vi "emballage nouvelle série_GPAO.vi"(1 "CodeBarFix":string, 2 "Nom du produit":string="12-216E-01-25 F120023 500mA 10Ohm", 3 "error in (no error)":errorcluster caption="entrée d'erreur (pas d'erreur)", 6 "Verif.Indice Client":bool) -> (5 "error out":errorcluster caption="sortie d'erreur", 11 "Indice Client":string, 14 "No commande FAS":string, 16 "DATA cmde":T1={"n°article FAS"="12-216E-01-25 F120023 500mA 10ohm", "n° cmde FAS"="R03844/08-01.01.01", "quantité cmde"="4", "ID LIG cmde"="225540", "n° cmde client"="120565              ", "nom client"="Fluid Automat. Systems GmbH", "n° article client"="21088", "indice revision client"="      ", "société de facturation"="FAS Medic SA                            ", "langue a utiliser"="ALL"}, 17 "Quantité de la commande":string="4", 18 "Commande interne":bool, 19 "Annuler(T=OK)":bool)   [LabVIEW 2020]
uses:
  Modules/FS/60_FS_Controles/60_FS_SetGet.ctl
  VG_VerifTests_ModeRetour.vi
panel:
  out "Cde_GPAO":bool
  in  "Cmde_Interne?":bool
  out "Indice Piece":string
  out "Tableau historique":string[][](array[string])=[["112105740008090004", "01.01.2001 01:01:00", "55", "01234/08-01.01.01", "1", "0"], ["112105740008090006", "01.01.2001 01:01:00", "55", "56789/08-01.01.01", "3", "0"], ["112105740008090007", "01.01.2001 01:01:00", "55", "56789/08-01.01.01", "4", "0"], ["112105740008090007", "01.01.2001 01:01:00", "55", "00123/08-01.01.01", "2", "1"]]
  out "Glissière 2":u8(slide)=100 caption="Identification terminé." scale=0.0..100.0
  in  "Valider qtté":bool
  in  "modifier qtté":bool
  in  "Numéro de commande FAS":string(combo)
  in  "Valider cmde":bool
  in  "Annuler?":bool
  # "La recherche se fait uniquement avec le numéro d'article et du numéro de file.\nLa designation (24V,...) n'est pas tenue compte (sauf pour les Flatprop) !!"
  # "Numéro de commande FAS"
  # "Seul un responsable peut valider une commande R (Retour)"
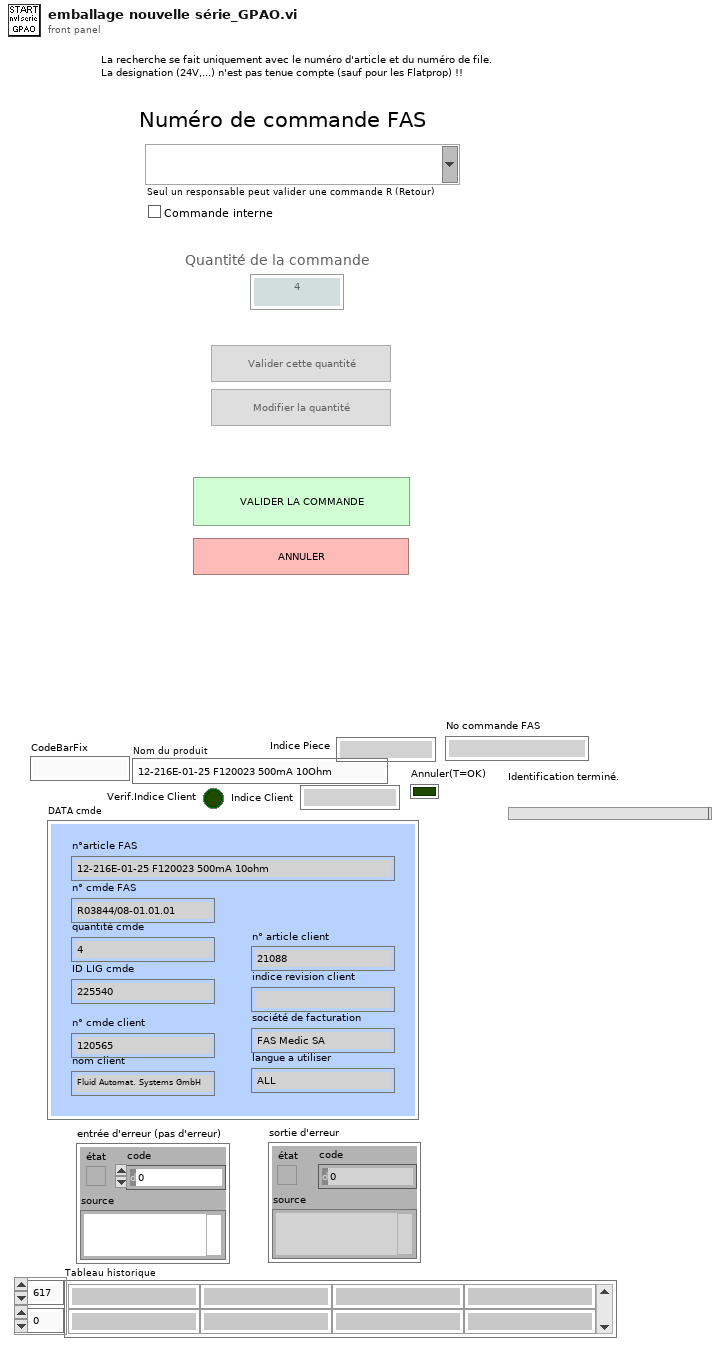
[diagram p1: front panel]
types:
  T1 = typedef "DATA commande.ctl" = cluster{"n°article FAS":string, "n° cmde FAS":string, "quantité cmde":string, "ID LIG cmde":string, "n° cmde client":string, "nom client":string, "n° article client":string, "indice revision client":string, "société de facturation":string, "langue a utiliser":string}
  T2 = typedef "60_FS_SetGet.ctl" = enum16{"set", "get"}
  T3 = enum16{"n° produit", "date", "opérateur", "n° cmde", "n° carton"}
  T4 = typedef "Emballage_BDD_param_Produit.ctl" = cluster{"No_Valve_FAS":string, "suffixe":string, "designation":string, "indice_produit":string, "code_barre_fixe":string, "affiche_code_barre_client":string, "affiche_no_client":string, "Nb_vlve_par_carton":u16, "melange_des_lots_possible":string, "id_article":string, "Indice_Rev":string, "Famille":string, "date":string, "code_barre_fixe_Fin":string, "Longeur_No_Serie":string}
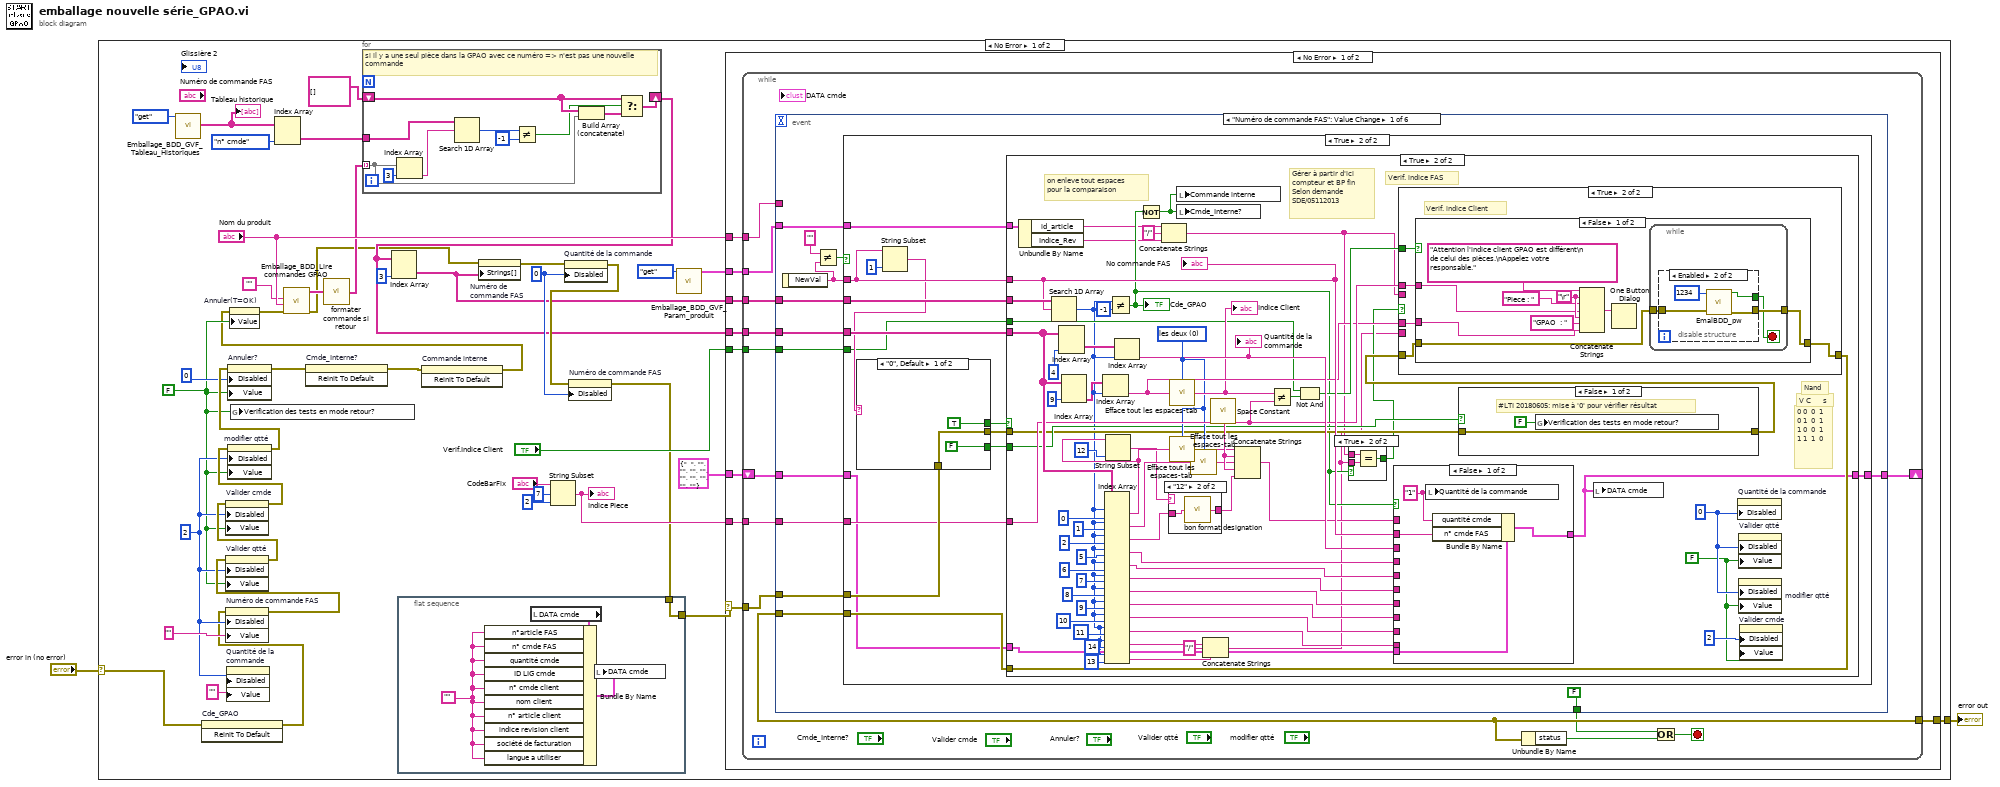
[diagram p0: block diagram]
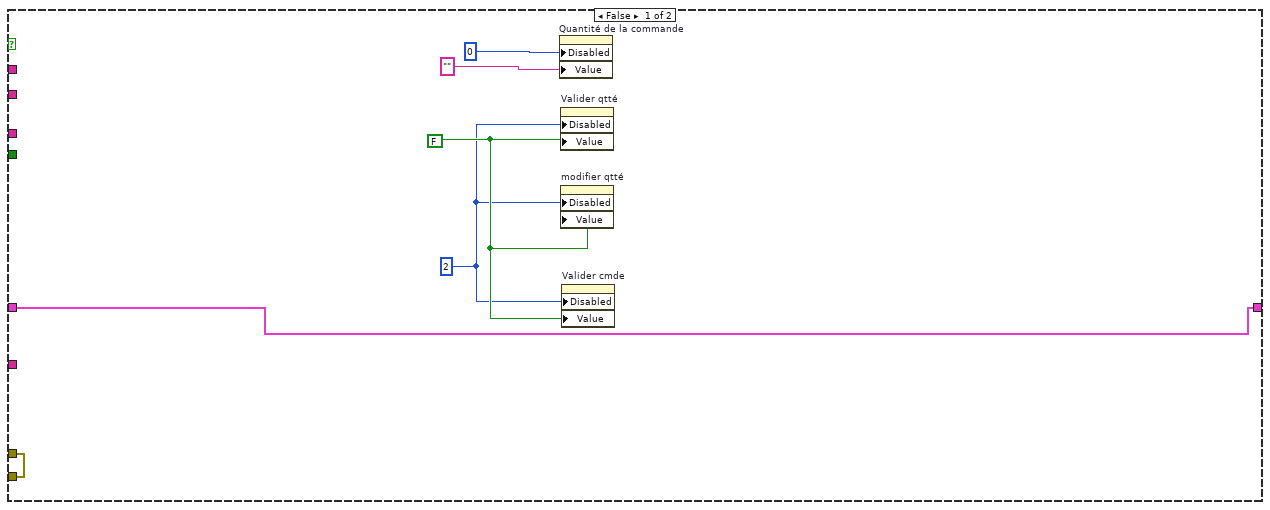
[diagram p2: hidden frame]
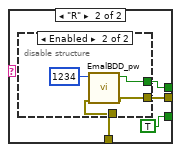
[diagram p3: hidden frame]
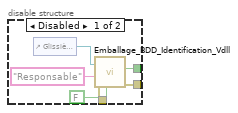
[diagram p4: hidden frame]
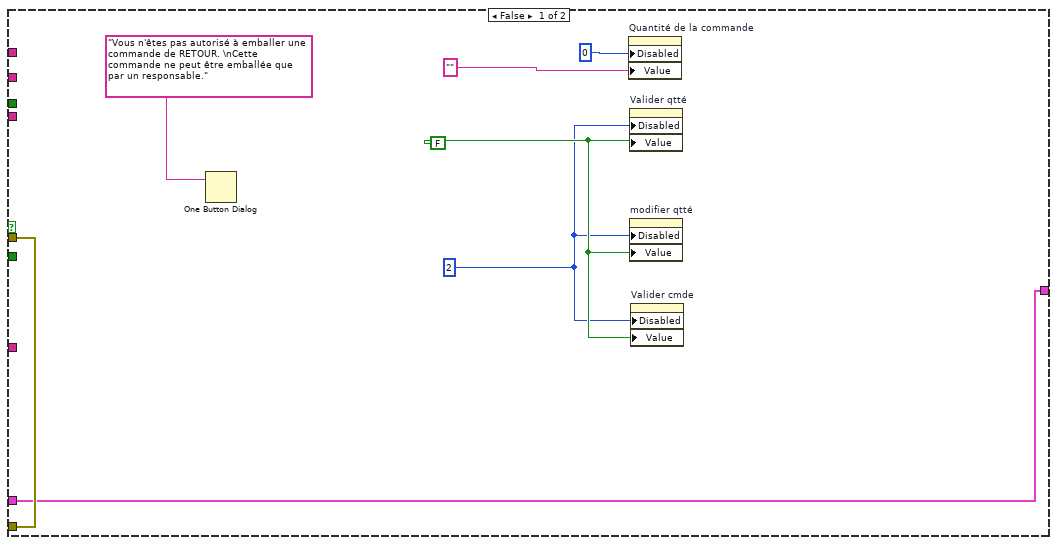
[diagram p5: hidden frame]
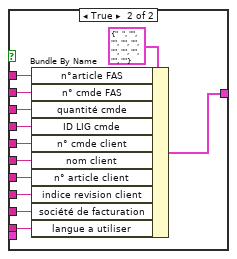
[diagram p6: hidden frame]
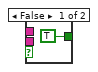
[diagram p7: hidden frame]
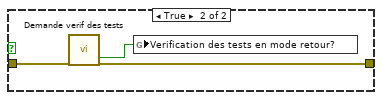
[diagram p8: hidden frame]
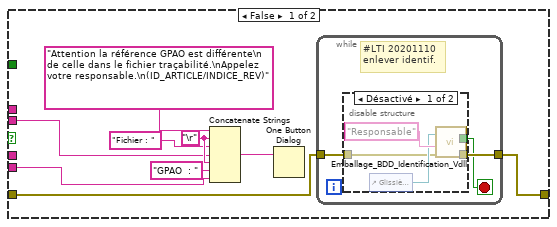
[diagram p9: hidden frame]
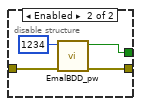
[diagram p10: hidden frame]
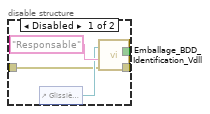
[diagram p11: hidden frame]
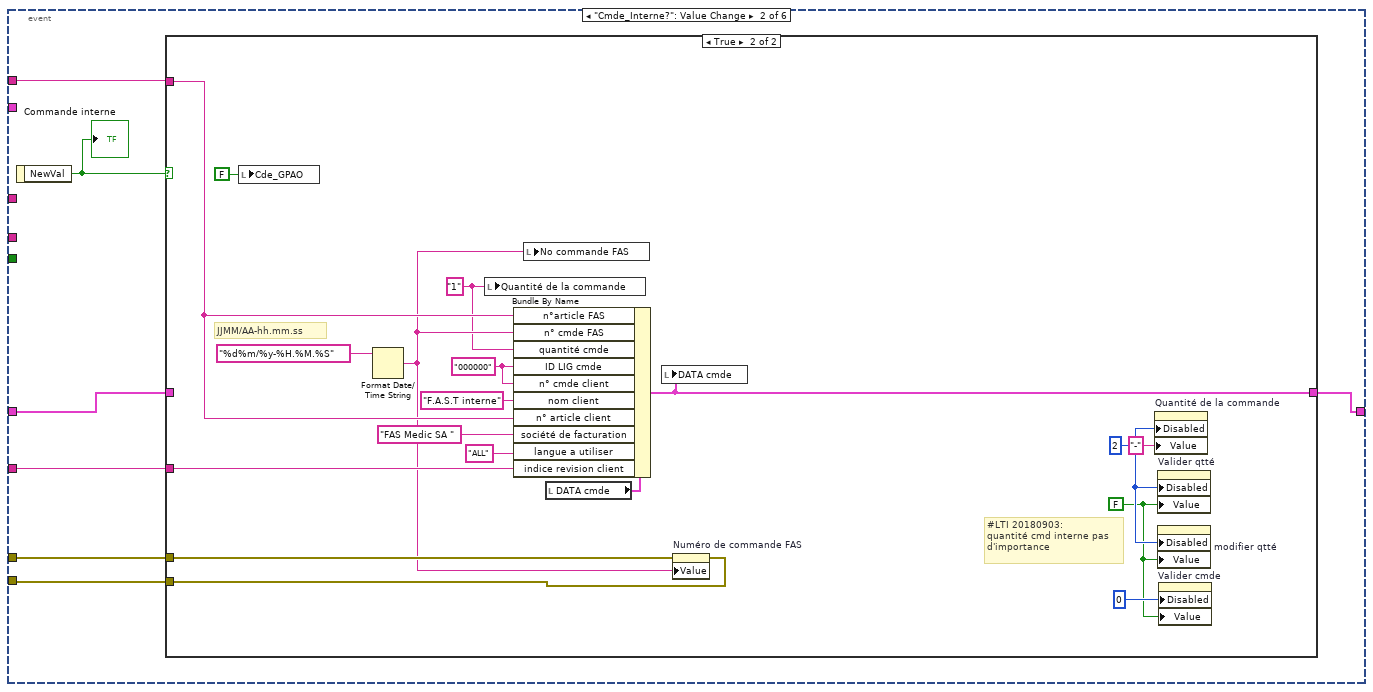
[diagram p14: hidden frame]
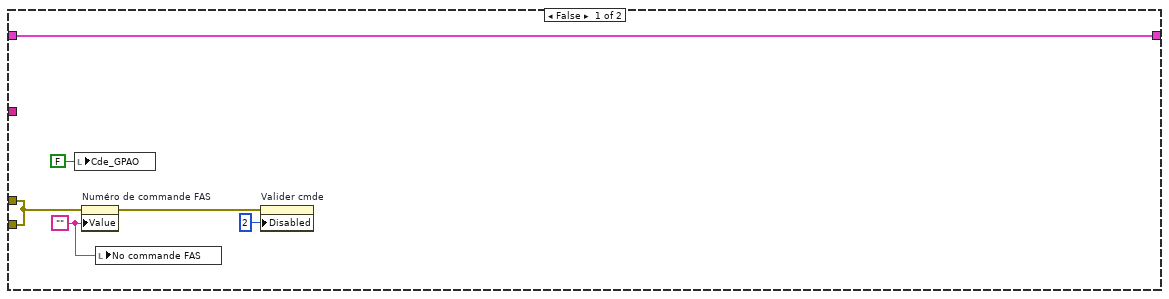
[diagram p15: hidden frame]
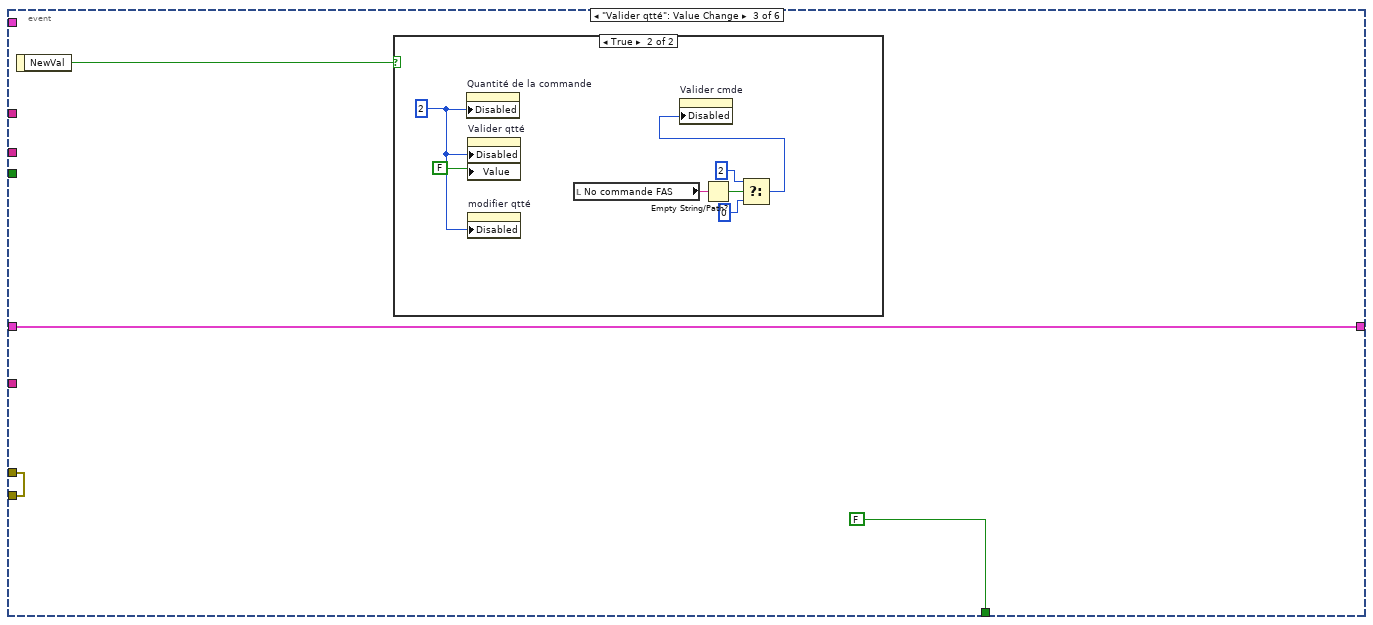
[diagram p16: hidden frame]
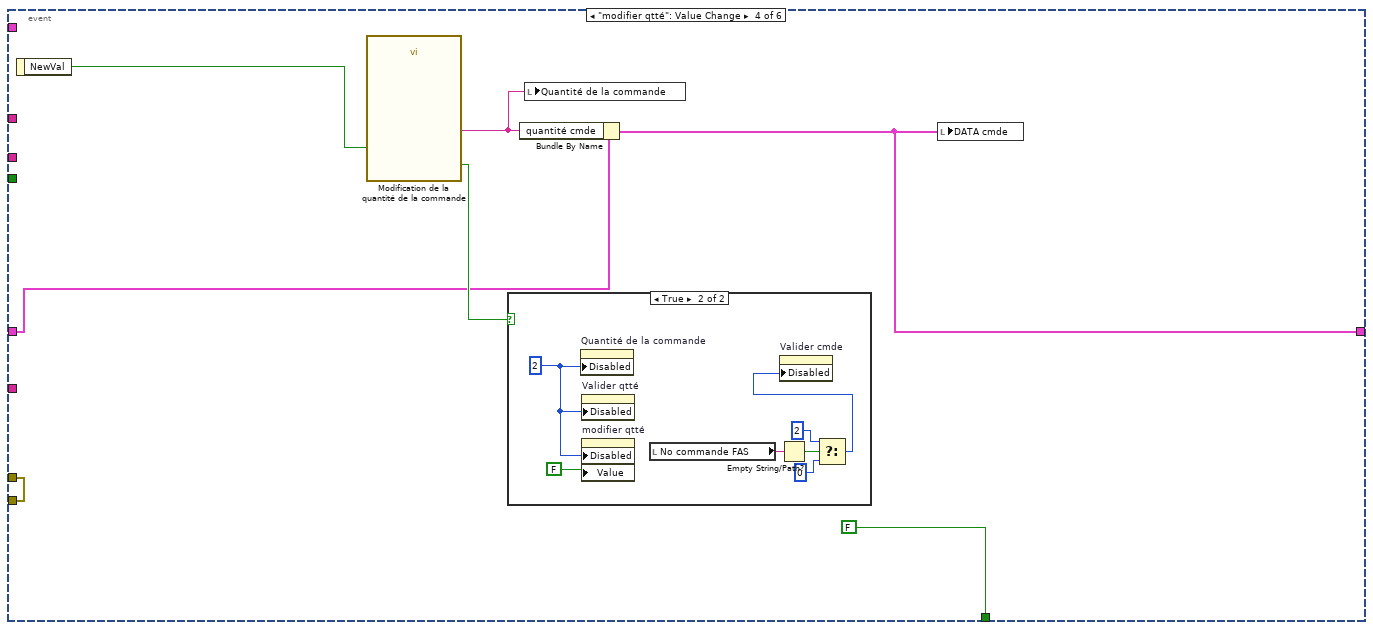
[diagram p18: hidden frame]
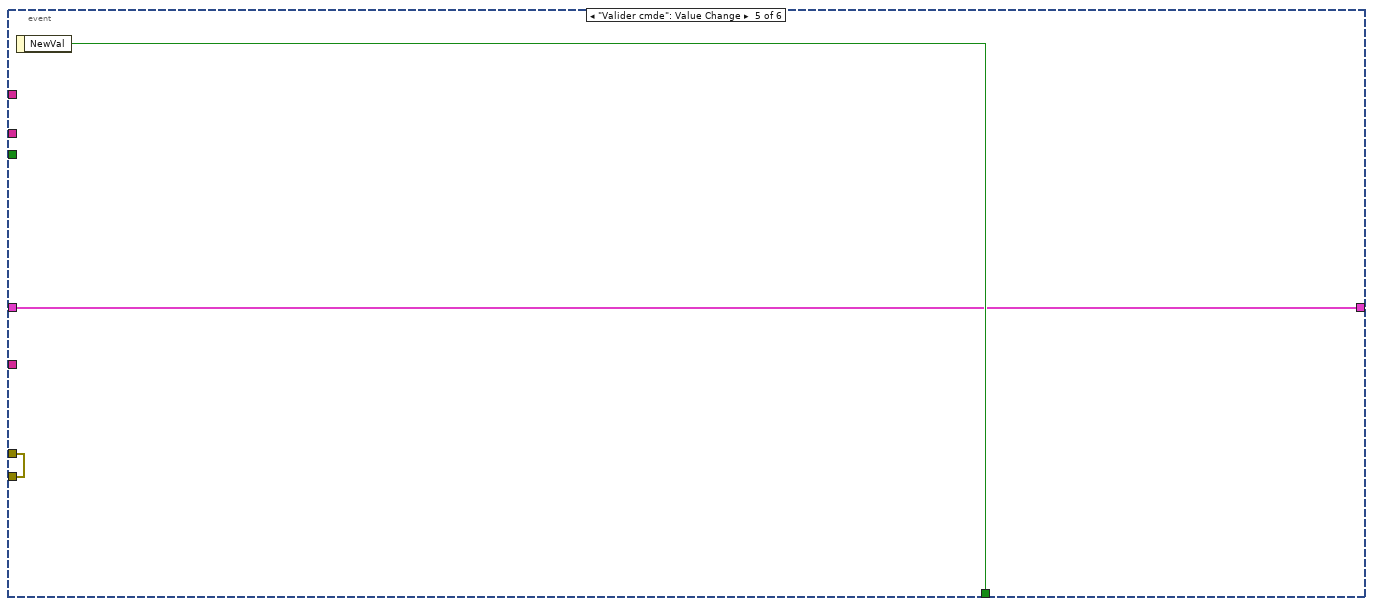
[diagram p20: hidden frame]
diagram:
  n1 = case shown="No Error" "error in (no error)" {
    selector: "error in (no error)" -> [w9 w350]
    tunnel: [w29 w350] -> w1
    frame No Error {
      w35 = u8 0 ("Désactivé")
      w39 = u8 2 ("Désactivé")
      w14 = FALSE
      n2 = call "Emballage_BDD_GVF_Tableau_Historiques.vi"("SetGet"=60_FS_SetGet."get") -> ("Tableau historique OUT"=w6:string[][])  [unwired: 9 in, 1 out]
      "Tableau historique" <- w6
      n3 = invoke on="Cde_GPAO" class="Bool (strict)" method="Reinit To Default"(error in=w9) -> (error out=w8:errorcluster)  [unwired: 2 in, 2 out]
      n4 = property on="Numéro de commande FAS" class="CmbBox"(error in=w8, "Disabled"=w39, "Value"="" ("Numéro de commande FAS")) -> (error out=w44:errorcluster)  [unwired: 1 in, 1 out]
      n5 = property on="Valider qtté" class="Bool (strict)"(error in=w44, "Disabled"=w39, "Value"=w14) -> (error out=w43:errorcluster)  [unwired: 1 in, 1 out]
      n6 = property on="Valider cmde" class="Bool (strict)"(error in=w43, "Disabled"=w39, "Value"=w14) -> (error out=w41:errorcluster)  [unwired: 1 in, 1 out]
      n7 = property on="Quantité de la commande" class="Str"("Disabled"=w39, "Value"="" ("Quantité de la commande")) -> ()  [unwired: 2 in, 2 out]
      n8 = property on="modifier qtté" class="Bool (strict)"(error in=w41, "Disabled"=w39, "Value"=w14) -> (error out=w40:errorcluster)  [unwired: 1 in, 1 out]
      n9 = property on="Annuler?" class="Bool (strict)"(error in=w40, "Disabled"=u8 0 ("Désactivé"), "Value"=w14) -> (error out=w13:errorcluster)  [unwired: 1 in, 1 out]
      n10 = global write "VG_VerifTests_ModeRetour.vi" "Verification des tests en mode retour?"(w14) -> ()
      n11 = Index Array(array=w6, index (col)=T3."n° cmde" ("Filtre")) -> (element=w26:string[])  [unwired: 1 in]
      n12 = invoke on="Cmde_Interne?" class="Bool (strict)" method="Reinit To Default"(error in=w13) -> (error out=w12:errorcluster)  [unwired: 2 in, 2 out]
      n13 = flat-sequence {
        tunnel: w10 -> [w345]
        tunnel: [w345] -> w30
        frame #0 {
          w344 = ""
          n14 = local read "DATA cmde"() -> (w347:T1)
          n15 = Bundle By Name(cluster=w347, "n°article FAS"=w344, "n° cmde FAS"=w344, "quantité cmde"=w344, "ID LIG cmde"=w344, "n° cmde client"=w344, "nom client"=w344, "n° article client"=w344, "indice revision client"=w344, "société de facturation"=w344, "langue a utiliser"=w344) -> (w346:T1)
          n16 = local write "DATA cmde"(w346) -> ()
        }
      }
      n17 = invoke on="Commande interne" class="Bool (strict)" method="Reinit To Default"(error in=w12) -> (error out=w11:errorcluster)  [unwired: 2 in, 2 out]
      n18 = property on="Annuler(T=OK)" class="Bool (strict)"(error in=w11, "Value"=w14) -> (error out=w33:errorcluster)  [unwired: 1 in, 1 out]
      n19 = call "Emballage_BDD_Lire  commandes GPAO.vi"("error in"=w33, "article"="Nom du produit", "Numéro commande"="") -> ("error out"=w21:errorcluster, "Tab cmde GPAO"=w31:string[][])  [unwired: 3 in, 4 out]
      n20 = call "formater commande si retour.vi"("Tab cmde GPAO IN"=w31) -> ("Tab cmde GPAO OUT"=w24:string[][])
      n21 = for {
        tunnel: w26 -> [w49]
        shift-right: [w54] -> w22
        shift-left: string[][] [] -> [w53]
        tunnel: w24 -> [w50] mode=indexing
        # "si il y a une seul pièce dans la GPAO avec ce numéro => n'est pas une nouvelle\ncommande"
        n22 = Index Array(array=w50, index=3 ("indice désactivé (col)")) -> (element=w48:string)
        n23 = Search 1D Array(1D array=w49, element=w48) -> (index of element=w47:i32)  [unwired: 1 in]
        n24 = Not Equal?(x=w47, y=-1) -> (x != y?=w45:bool)
        n25 = Build Array (concatenate)(w53, w50) -> (w52:string[][])
        n26 = Select(t=w53, s=w45, f=w52) -> (s? t:f=w54:string[][])
      }
      n27 = Index Array(array=w22, index (col)=3 ("indice désactivé (col)")) -> (element=w23:string[])  [unwired: 1 in]
      n28 = property on="Numéro de \ncommande FAS" class="CmbBox"(error in=w21, "Strings[]"=w23) -> (error out=w36:errorcluster)  [unwired: 1 in, 1 out]
      n29 = String Subset(string="CodeBarFix", offset (0)=7, length (rest)=2 ("longueur (reste)")) -> (substring=w16:string)
      "Indice Piece" <- w16
      n30 = property on="Quantité de la commande" class="Str"(error in=w36, "Disabled"=w35) -> (error out=w37:errorcluster)  [unwired: 1 in, 1 out]
      n31 = property on="Numéro de commande FAS" class="CmbBox"(error in=w37, "Disabled"=w35) -> (error out=w10:errorcluster)  [unwired: 1 in, 1 out]
      n32 = call "Emballage_BDD_GVF_Param_produit.vi"("Énum"=enum16{"set", "get"}."get") -> ("CLS_param_produit"=w3:T4)  [unwired: 7 in, 3 out]
      n33 = case shown="No Error" w30 {
        selector: w30 -> [w60 w343]
        tunnel: w23 -> [w63 _]
        tunnel: w22 -> [w62 _]
        tunnel: [w61 w343] -> w29
        tunnel: "Nom du produit" -> [w59 _]
        tunnel: w16 -> [w58 _]
        tunnel: "Verif.Indice Client" -> [w57 _]
        tunnel: T1 {"n°article FAS"="  ", "n° cmde FAS"="", "quantité cmde"="", "ID LIG cmde"="", "n° cmde client"="", "nom client"="", "n° article client"="", "indice revision client"="", "société de facturation"="", "langue a utiliser"=""} ("DATA cmde") -> [w56 _]
        tunnel: w3 -> [w55 _]
        frame No Error {
          n34 = while {
            tunnel: w63 -> [w76]
            tunnel: w62 -> [w75]
            tunnel: [w72] -> w61
            tunnel: w60 -> [w73]
            tunnel: w59 -> [w74]
            tunnel: w58 -> [w68]
            tunnel: w57 -> [w67]
            shift-right: [w66] -> _
            shift-left: w56 -> [w65]
            tunnel: w55 -> [w64]
            stop <- w71 stop-if-true
            n35 = event shown="[0] \"Numéro de commande FAS\": Value Change" {
              selector: _ -> [_ _ _ _ _ _]
              dyn-events: _ -> [_ _ _ _ _ _]
              timeout: _ -> [_ _ _ _ _ _]
              tunnel: w76 -> [w89 _ _ _ _ _]
              tunnel: w75 -> [w87 _ _ _ _ _]
              tunnel: [FALSE _ FALSE FALSE w336 w340] -> w70
              tunnel: w74 -> [_ w281 _ _ _ _]
              tunnel: w73 -> [w83 w283 w310 w322 w335 w338]
              tunnel: [w82 w282 w310 w322 w335 w338] -> w72
              tunnel: w68 -> [w81 w280 _ _ _ _]
              tunnel: w67 -> [w80 _ _ _ _ _]
              tunnel: [w79 w279 w309 w320 w334 w337] -> w66
              tunnel: w65 -> [w78 w278 w309 w321 w334 _]
              tunnel: w64 -> [w77 _ _ _ _ _]
              event "Numéro de commande FAS": Value Change {
                n36 = event-data() -> ("NewVal"=w84:string)  [unwired: 1 in]
                n37 = Not Equal?(x="" ("nouvel élément/sous-tableau"), y=w84) -> (x != y?=w86:bool)
                n38 = case shown="True" w86 {
                  tunnel: w89 -> [_ w110]
                  tunnel: w84 -> [_ w108]
                  tunnel: w87 -> [_ w109]
                  tunnel: w83 -> [w91 w104]
                  tunnel: [w91 w102] -> w82
                  tunnel: w81 -> [_ w101]
                  tunnel: w80 -> [_ w100]
                  tunnel: [w90 w98] -> w79
                  tunnel: w78 -> [w90 w97]
                  tunnel: w77 -> [_ w96]
                  frame False {
                    w95 = FALSE
                    w92 = u8 2 ("Désactivé")
                    n39 = property on="Quantité de la commande" class="Str"("Disabled"=u8 0 ("Désactivé"), "Value"="" ("nouvel élément/sous-tableau")) -> ()  [unwired: 2 in, 2 out]
                    n40 = property on="Valider qtté" class="Bool (strict)"("Disabled"=w92, "Value"=w95) -> ()  [unwired: 2 in, 2 out]
                    n41 = property on="modifier qtté" class="Bool (strict)"("Disabled"=w92, "Value"=w95) -> ()  [unwired: 2 in, 2 out]
                    n42 = property on="Valider cmde" class="Bool (strict)"("Disabled"=w92, "Value"=w95) -> ()  [unwired: 2 in, 2 out]
                  }
                  frame True {
                    n43 = String Subset(string=w108, length (rest)=1 ("longueur (reste)")) -> (substring=w106:string)  [unwired: 1 in]
                    n44 = case shown="\"0\", Default" w106 {
                      tunnel: [TRUE w116] -> w105
                      tunnel: w104 -> [w112 w117]
                      tunnel: [w112 w115] -> w103
                      tunnel: [FALSE ("lecture seul possible ?") TRUE ("lecture seul possible ?")] -> w99
                      frame "0", Default {
                      }
                      frame "R" {
                        n45 = disable-structure shown="Enabled" {
                          disable-tunnel: w117 -> [w121 w126]
                          disable-tunnel: [w120 w125] -> w116
                          disable-tunnel: [w118 w127] -> w115
                          frame Disabled {
                            n46 = control-ref of="Glissière 2"() -> (w119:refnum<vi>)
                            n47 = call "Emballage_BDD_Identification_Vdll.vi"("Glissière"=w119, "lecture seul possible ?"=FALSE, "error in"=w121, "Posage choisi"="Responsable") -> ("error Out"=w118:errorcluster, "OK"=w120:bool)  [unwired: 3 in, 3 out]
                          }
                          frame Enabled {
                            n48 = call "EmalBDD_pw.vi"("Error in"=w126, "PWattendu"=u32 1234) -> ("Error Out"=w127:errorcluster, "pwOK?"=w125:bool)  [unwired: 8 in]
                          }
                        }
                      }
                    }
                    n49 = case shown="True" w105 {
                      tunnel: w110 -> [_ w201]
                      tunnel: w108 -> [_ w193]
                      tunnel: w109 -> [_ w165]
                      tunnel: w103 -> [w129 w154]
                      tunnel: [w129 w166] -> w102
                      tunnel: w101 -> [_ w160]
                      tunnel: w100 -> [_ w147]
                      tunnel: w99 -> [_ w155]
                      tunnel: [w128 w150] -> w98
                      tunnel: w97 -> [w128 w149]
                      tunnel: w96 -> [_ w146]
                      frame False {
                        w133 = FALSE
                        w130 = u8 2 ("Désactivé")
                        n50 = One Button Dialog(message="Vous n'êtes pas autorisé à emballer une commande de RETOUR. \nCette commande ne peut être emballée que par un responsable.") -> ()  [unwired: 1 in, 1 out]
                        n51 = property on="Quantité de la commande" class="Str"("Disabled"=u8 0 ("Désactivé"), "Value"="" ("nouvel élément/sous-tableau")) -> ()  [unwired: 2 in, 2 out]
                        n52 = property on="Valider qtté" class="Bool (strict)"("Disabled"=w130, "Value"=w133) -> ()  [unwired: 2 in, 2 out]
                        n53 = property on="modifier qtté" class="Bool (strict)"("Disabled"=w130, "Value"=w133) -> ()  [unwired: 2 in, 2 out]
                        n54 = property on="Valider cmde" class="Bool (strict)"("Disabled"=w130, "Value"=w133) -> ()  [unwired: 2 in, 2 out]
                      }
                      frame True {
                        w157 = u16 0 items=["les deux", "début de la chaîne", "fin de chaîne"] ("location (both)")
                        w185 = FALSE
                        w189 = u8 0 ("Désactivé")
                        # "Gérer à partir d'ici \ncompteur et BP fin\nSelon demande \nSDE/05112013"
                        # "Nand"
                        # "V C      s"
                        # "0 0  0  1\n0 1  0  1\n1 0  0  1\n1 1  1  0"
                        # "Verif. indice FAS"
                        # "on enleve tout espaces \npour la comparaison"
                        n55 = Unbundle By Name(w146) -> ("id_article"=w144:string, "Indice_Rev"=w138:string)
                        n56 = Search 1D Array(1D array=w201, element=w193) -> (index of element=w141:i32)  [unwired: 1 in]
                        n57 = Index Array(array=w165, index (col)=4 ("indice désactivé (col)")) -> (element=w186:string[])  [unwired: 1 in]
                        n58 = Index Array(array=w165, index (col)=9 ("indice désactivé (col)")) -> (element=w163:string[])  [unwired: 1 in]
                        n59 = Index Array(array=w163, index=w141) -> (element=w159:string)
                        n60 = Index Array(array=w165, index (row) #1=w141, index (col) #1=0 ("indice désactivé (col)"), index (row) #2=w141, index (col) #2=1 ("indice désactivé (col)"), index (row) #3=w141, index (col) #3=2 ("indice désactivé (col)"), index (row) #4=w141, index (col) #4=5 ("indice désactivé (col)"), index (row) #5=w141, index (col) #5=6 ("indice désactivé (col)"), index (row) #6=w141, index (col) #6=7 ("indice désactivé (col)"), index (row) #7=w141, index (col) #7=8 ("indice désactivé (col)"), index (row) #8=w141, index (col) #8=9 ("indice désactivé (col)"), index (row) #9=w141, index (col) #9=10 ("indice désactivé (col)"), index (row) #10=w141, index (col) #10=11 ("indice désactivé (col)"), index (row) #11=w141, index (col) #11=14 ("indice (col)"), index (row) #12=w141, index (col) #12=13 ("indice (col)")) -> (element #1=w171:string, element #2=w179:string, element #3=w168:string, element #4=w191:string, element #5=w190:string, element #6=w177:string, element #7=w176:string, element #8=w175:string, element #9=w174:string, element #10=w173:string, element #11=w143:string, element #12=w136:string)
                        n61 = String Subset(string=w171, length (rest)=12 ("longueur (reste)")) -> (substring=w169:string)  [unwired: 1 in]
                        n62 = Not Equal?(x=w141, y=-1) -> (x != y?=w148:bool)
                        "Cde_GPAO" <- w148
                        n63 = Index Array(array=w186, index=w141) -> (element=w192:string)
                        "Quantité de la commande" <- w192
                        n64 = Not(x=w148) -> (.not. x?=w151:bool)
                        n65 = Concatenate Strings(w144, "/" ("chaîne"), w138) -> (w140:string)
                        n66 = case shown="\"12\"" w169 {
                          tunnel: [w275 w277] -> w172
                          tunnel: w168 -> [w275 w276]
                          frame Default {
                          }
                          frame "12" {
                            n67 = call "bon format designation.vi"("Chaîne IN"=w276) -> ("Chaîne OUT"=w277:string)
                          }
                        }
                        n68 = call "Efface tout les espaces-tab.vi"("string"=w159, "location (both)"=w157) -> ("trimmed string"=w158:string)
                        "Indice Client" <- w158
                        n69 = call "Efface tout les espaces-tab.vi"("string"=w171, "location (both)"=w157) -> ("trimmed string"=w180:string)
                        n70 = local write "Commande interne"(w151) -> ()
                        n71 = local write "Cmde_Interne?"(w151) -> ()
                        n72 = call "Efface tout les espaces-tab.vi"("string"=w179, "location (both)"=w157) -> ("trimmed string"=w178:string)
                        n73 = Concatenate Strings(w143, "/" ("chaîne"), w136) -> (w137:string)
                        n74 = call <vilib>:"Space Constant.vi"() -> ("String"=w181:string)
                        n75 = Concatenate Strings(w180, w181, w178, w181, w172) -> (w167:string)
                        n76 = Not Equal?(x=w158, y=w160) -> (x != y?=w162:bool)
                        n77 = Not And(1:w162, 2:w147) -> (0:w161:bool)
                        n78 = case shown="True" w148 {
                          tunnel: w140 -> [_ w221]
                          tunnel: w137 -> [_ w220]
                          tunnel: [TRUE w219] -> w153
                          frame False {
                          }
                          frame True {
                            n79 = Equal?(x=w221, y=w220) -> (x = y?=w219:bool)
                          }
                        }
                        n80 = case shown="False" w148 {
                          tunnel: w193 -> [w205 w217]
                          tunnel: w192 -> [_ w216]
                          tunnel: w191 -> [_ w215]
                          tunnel: w190 -> [_ w214]
                          tunnel: w177 -> [_ w213]
                          tunnel: w176 -> [_ w212]
                          tunnel: w175 -> [_ w211]
                          tunnel: w174 -> [_ w210]
                          tunnel: w173 -> [_ w209]
                          tunnel: w167 -> [_ w208]
                          tunnel: [w203 w206] -> w150
                          tunnel: w149 -> [w204 _]
                          frame False {
                            w202 = "1" ("Quantité de la commande")
                            n81 = local write "Quantité de la commande"(w202) -> ()
                            n82 = Bundle By Name(cluster=w204, "quantité cmde"=w202, "n° cmde FAS"=w205) -> (w203:T1)
                          }
                          frame True {
                            n83 = Bundle By Name(cluster=T1 {"n°article FAS"="  ", "n° cmde FAS"="", "quantité cmde"="", "ID LIG cmde"="", "n° cmde client"="", "nom client"="", "n° article client"="", "indice revision client"="", "société de facturation"="", "langue a utiliser"=""} ("DATA cmde"), "n°article FAS"=w208, "n° cmde FAS"=w217, "quantité cmde"=w216, "ID LIG cmde"=w215, "n° cmde client"=w214, "nom client"=w213, "n° article client"=w212, "indice revision client"=w211, "société de facturation"=w210, "langue a utiliser"=w209) -> (w206:T1)
                          }
                        }
                        n84 = case shown="False" w155 {
                          tunnel: w154 -> [w223 w226]
                          tunnel: [w223 w225] -> w156
                          frame False {
                            # "#LTI 20180605: mise à '0' pour vérifier résultat"
                            n85 = global write "VG_VerifTests_ModeRetour.vi" "Verification des tests en mode retour?"(FALSE ("Verification des tests en mode retour?")) -> ()
                          }
                          frame True {
                            n86 = call "Demande verif des tests"("error in (no error)"=w226) -> ("OUI"=w224:bool, "error out"=w225:errorcluster)  [unwired: 17 in]
                            n87 = global write "VG_VerifTests_ModeRetour.vi" "Verification des tests en mode retour?"(w224) -> ()
                          }
                        }
                        n88 = case shown="True" w153 {
                          tunnel: w140 -> [w232 _]
                          tunnel: w137 -> [w230 _]
                          tunnel: w156 -> [w228 w252]
                          tunnel: [w227 w251] -> w166
                          tunnel: w159 -> [_ w250]
                          tunnel: w160 -> [_ w249]
                          tunnel: w161 -> [_ w248]
                          frame False {
                            w233 = "\r"
                            n89 = Concatenate Strings("Attention la référence GPAO est différente\n de celle dans le fichier traçabilité.\nAppelez votre responsable.\n(ID_ARTICLE/INDICE_REV)" ("message"), w233, "Fichier : " ("chaîne"), w232, w233, "GPAO  : " ("chaîne"), w230) -> (w235:string)
                            n90 = One Button Dialog(message=w235) -> ()  [unwired: 1 in, 1 out]
                            n91 = while {
                              tunnel: w228 -> [w238]
                              tunnel: [w237] -> w227
                              stop <- w236 stop-if-true
                              # "#LTI 20201110\nenlever identif."
                              n92 = disable-structure shown="Désactivé" {
                                disable-tunnel: w238 -> [w241 w246]
                                disable-tunnel: [w240 w245] -> w237
                                disable-tunnel: [w239 w244] -> w236
                                frame Disabled {
                                n93 = control-ref of="Glissière 2"() -> (w242:refnum<vi>)
                                n94 = call "Emballage_BDD_Identification_Vdll.vi"("Glissière"=w242, "error in"=w241, "Posage choisi"="Responsable") -> ("error Out"=w240:errorcluster, "OK"=w239:bool)  [unwired: 4 in, 3 out]
                                }
                                frame Enabled {
                                n95 = call "EmalBDD_pw.vi"("Error in"=w246, "PWattendu"=u32 1234) -> ("Error Out"=w245:errorcluster, "pwOK?"=w244:bool)  [unwired: 8 in]
                                }
                              }
                            }
                          }
                          frame True {
                            # "Verif. indice Client"
                            n96 = case shown="False" w248 {
                              tunnel: w249 -> [w258 _]
                              tunnel: w250 -> [w256 _]
                              tunnel: w252 -> [w254 w274]
                              tunnel: [w253 w274] -> w251
                              frame False {
                                w259 = "\r"
                                n97 = Concatenate Strings("Attention l'indice client GPAO est différent\n de celui des pièces.\nAppelez votre responsable." ("message"), w259, "Piece : " ("chaîne"), w258, w259, "GPAO  : " ("chaîne"), w256) -> (w261:string)
                                n98 = One Button Dialog(message=w261) -> ()  [unwired: 1 in, 1 out]
                                n99 = while {
                                tunnel: w254 -> [w264]
                                tunnel: [w263] -> w253
                                stop <- w262 stop-if-true
                                n100 = disable-structure shown="Enabled" {
                                disable-tunnel: w264 -> [w267 w272]
                                disable-tunnel: [w266 w271] -> w263
                                disable-tunnel: [w265 w270] -> w262
                                frame Disabled {
                                n101 = control-ref of="Glissière 2"() -> (w268:refnum<vi>)
                                n102 = call "Emballage_BDD_Identification_Vdll.vi"("Glissière"=w268, "error in"=w267, "Posage choisi"="Responsable") -> ("error Out"=w266:errorcluster, "OK"=w265:bool)  [unwired: 4 in, 3 out]
                                }
                                frame Enabled {
                                n103 = call "EmalBDD_pw.vi"("Error in"=w272, "PWattendu"=u32 1234) -> ("Error Out"=w271:errorcluster, "pwOK?"=w270:bool)  [unwired: 8 in]
                                }
                                }
                                }
                              }
                              frame True {
                                # "pas de vérifs ou indices OK"
                              }
                            }
                          }
                        }
                        n104 = local write "DATA cmde"(w150) -> ()
                        n105 = property on="Quantité de la commande" class="Str"("Disabled"=w189) -> ()  [unwired: 2 in, 2 out]
                        n106 = property on="Valider qtté" class="Bool (strict)"("Disabled"=w189, "Value"=w185) -> ()  [unwired: 2 in, 2 out]
                        n107 = property on="modifier qtté" class="Bool (strict)"("Disabled"=w189, "Value"=w185) -> ()  [unwired: 2 in, 2 out]
                        n108 = property on="Valider cmde" class="Bool (strict)"("Disabled"=u8 2 ("Désactivé"), "Value"=w185) -> ()  [unwired: 2 in, 2 out]
                        "No commande FAS" <- w193
                      }
                    }
                  }
                }
              }
              event "Cmde_Interne?": Value Change {
                n109 = event-data() -> ("NewVal"=w284:bool)  [unwired: 1 in]
                "Commande interne" <- w284
                n110 = case shown="True" w284 {
                  tunnel: w283 -> [w290 w298]
                  tunnel: [w290 w297] -> w282
                  tunnel: w281 -> [_ w302]
                  tunnel: w280 -> [_ w299]
                  tunnel: [w287 w293] -> w279
                  tunnel: w278 -> [w287 _]
                  frame False {
                    w289 = ""
                    n111 = local write "Cde_GPAO"(FALSE ("Cde_GPAO")) -> ()
                    n112 = property on="Numéro de commande FAS" class="CmbBox"(error in=w290, "Value"=w289) -> (error out=w285:errorcluster)  [unwired: 1 in, 1 out]
                    n113 = local write "No commande FAS"(w289) -> ()
                    n114 = property on="Valider cmde" class="Bool (strict)"(error in=w285, "Disabled"=u8 2 ("Désactivé")) -> ()  [unwired: 1 in, 2 out]
                  }
                  frame True {
                    w292 = "1" ("Quantité de la commande")
                    w304 = "000000" ("ID LIG cmde")
                    w305 = FALSE
                    w307 = u8 2 ("Désactivé")
                    # "#LTI 20180903:\nquantité cmd interne pas \nd'importance"
                    # "JJMM/AA-hh.mm.ss"
                    n115 = local write "Cde_GPAO"(FALSE ("Cde_GPAO")) -> ()
                    n116 = Format Date/Time String(time format string (%c)="%d%m/%y-%H.%M.%S" ("chaîne de format de l'heure (%c)")) -> (date/time string=w295:string)  [unwired: 2 in]
                    n117 = local write "Quantité de la commande"(w292) -> ()
                    n118 = local write "No commande FAS"(w295) -> ()
                    n119 = local read "DATA cmde"() -> (w308:T1)
                    n120 = Bundle By Name(cluster=w308, "n°article FAS"=w302, "n° cmde FAS"=w295, "quantité cmde"=w292, "ID LIG cmde"=w304, "n° cmde client"=w304, "nom client"="F.A.S.T interne", "n° article client"=w302, "société de facturation"="FAS Medic SA ", "langue a utiliser"="ALL", "indice revision client"=w299) -> (w293:T1)
                    n121 = local write "DATA cmde"(w293) -> ()
                    n122 = property on="Numéro de commande FAS" class="CmbBox"(error in=w298, "Value"=w295) -> (error out=w297:errorcluster)  [unwired: 1 in, 1 out]
                    n123 = property on="Quantité de la commande" class="Str"("Disabled"=w307, "Value"="-" ("Quantité de la commande")) -> ()  [unwired: 2 in, 2 out]
                    n124 = property on="Valider qtté" class="Bool (strict)"("Disabled"=w307, "Value"=w305) -> ()  [unwired: 2 in, 2 out]
                    n125 = property on="modifier qtté" class="Bool (strict)"("Disabled"=w307, "Value"=w305) -> ()  [unwired: 2 in, 2 out]
                    n126 = property on="Valider cmde" class="Bool (strict)"("Disabled"=u8 0 ("Désactivé"), "Value"=w305) -> ()  [unwired: 2 in, 2 out]
                  }
                }
              }
              event "Valider qtté": Value Change {
                n127 = event-data() -> ("NewVal"=w312:bool)  [unwired: 1 in]
                n128 = case shown="True" w312 {
                  frame False {
                  }
                  frame True {
                    w319 = u8 2 ("Désactivé")
                    n129 = property on="Quantité de la commande" class="Str"("Disabled"=w319) -> ()  [unwired: 2 in, 2 out]
                    n130 = property on="Valider qtté" class="Bool (strict)"("Disabled"=w319, "Value"=FALSE ("Valider qtté")) -> ()  [unwired: 2 in, 2 out]
                    n131 = property on="modifier qtté" class="Bool (strict)"("Disabled"=w319) -> ()  [unwired: 2 in, 2 out]
                    n132 = local read "No commande FAS"() -> (w317:string)
                    n133 = Empty String/Path?(string/path=w317) -> (empty?=w316:bool)
                    n134 = Select(t=u8 2 ("Désactivé"), s=w316, f=u8 0 ("Désactivé")) -> (s? t:f=w313:u8)
                    n135 = property on="Valider cmde" class="Bool (strict)"("Disabled"=w313) -> ()  [unwired: 2 in, 2 out]
                  }
                }
              }
              event "modifier qtté": Value Change {
                n136 = event-data() -> ("NewVal"=w324:bool)  [unwired: 1 in]
                n137 = call "Modification de la quantité de la commande"("Enable"=w324) -> ("Nouvelle quantité :"=w325:string, "OK"=w323:bool)  [unwired: 16 in, 1 out]
                n138 = case shown="True" w323 {
                  frame False {
                  }
                  frame True {
                    w333 = u8 2 ("Désactivé")
                    n139 = property on="Quantité de la commande" class="Str"("Disabled"=w333) -> ()  [unwired: 2 in, 2 out]
                    n140 = property on="Valider qtté" class="Bool (strict)"("Disabled"=w333) -> ()  [unwired: 2 in, 2 out]
                    n141 = property on="modifier qtté" class="Bool (strict)"("Disabled"=w333, "Value"=FALSE ("modifier qtté")) -> ()  [unwired: 2 in, 2 out]
                    n142 = local read "No commande FAS"() -> (w331:string)
                    n143 = Empty String/Path?(string/path=w331) -> (empty?=w330:bool)
                    n144 = Select(t=u8 2 ("Désactivé"), s=w330, f=u8 0 ("Désactivé")) -> (s? t:f=w327:u8)
                    n145 = property on="Valider cmde" class="Bool (strict)"("Disabled"=w327) -> ()  [unwired: 2 in, 2 out]
                  }
                }
                n146 = Bundle By Name(cluster=w321, "quantité cmde"=w325) -> (w320:T1)
                n147 = local write "Quantité de la commande"(w325) -> ()
                n148 = local write "DATA cmde"(w320) -> ()
              }
              event "Valider cmde": Value Change {
                n149 = event-data() -> ("NewVal"=w336:bool)  [unwired: 1 in]
              }
              event "Annuler?": Value Change {
                w337 = T1 {"n°article FAS"="  ", "n° cmde FAS"="", "quantité cmde"="", "ID LIG cmde"="", "n° cmde client"="", "nom client"="", "n° article client"="", "indice revision client"="", "société de facturation"="", "langue a utiliser"=""}  # DATA cmde
                n150 = event-data() -> ("NewVal"=w340:bool)  [unwired: 1 in]
                "Annuler(T=OK)" <- w340
                n151 = property on="Numéro de commande FAS" class="CmbBox"(error in=w338, "Value"="") -> ()  [unwired: 1 in, 2 out]
              }
            }
            n152 = Unbundle By Name(w72) -> ("status"=w69:bool)
            n153 = Or(x=w70, y=w69) -> (x .or. y?=w71:bool)
          }
        }
        frame Error {
          n154 = call "03_FS_GFV_Logfile.vi"("Chaîne"="Erreur Après initialisation de la liste des N° commandes", "States"=60_FS_SetGet."set") -> ()  [unwired: 8 in, 2 out]
        }
      }
    }
    frame Error {
      n155 = call "03_FS_GFV_Logfile.vi"("Chaîne"="Erreur avant nouvelle serie_GPAO", "States"=60_FS_SetGet."set") -> ()  [unwired: 8 in, 2 out]
    }
  }
  "error out" <- w1
